vi "SubPanel_DataCollection_Rev11_v11.vi"(0 "DCPowerInformationClusterArray_Input":T7(array[cluster]), 1 "VISAPowerInfoInputArray":T6(array[cluster]), 2 "Run Data SubPanel Input":T5, 4 "Oscilloscope Info Array":T4(array[cluster]) {"vertical coupling" items=["AC", "DC", "Ground"]}, 6 "New Run?":bool, 7 "error in":errorcluster) -> (20 "DCPowerInformationClusterArray_Output":T7(array[cluster]), 21 "VISAPowerInfoInputOutput":T6(array[cluster]), 22 "Run Data SubPanel Output":T5, 23 "RF Block Parameters Output":T1, 24 "Oscilloscope Info Array Output":T4(array[cluster]) {"vertical coupling" items=["AC", "DC", "Ground"]}, 25 "Reinitialize?":bool, 26 "Data Was Collected?":bool, 27 "error out":errorcluster)   [LabVIEW 2019]
uses:
  Controls/DataBlockControl.ctl
  Controls/QueueDataControl_V3.ctl
  <vilib>/Utility/file.llb/Write Delimited Spreadsheet (string).vi
  Controls/RFBlockControl.ctl
  <instrlib>/niScope/Controls/niScope vertical coupling.ctl
panel:
  in  "RF Block Input Array":T1[](array[typedef])
  out "RFSourceInfoArray":string[][](array[string])
  out "OscilloscopeInfoArray":string[][](array[string])
  out "Voltage Waveform Array":waveform(dbl)[](array[waveform])
  out "Current Waveform Array":waveform(dbl)[](array[waveform])
  out "Current Measurements Live":T2(graph)
  out "Voltage Measurements Live":T2(graph)
  out "DCPowerInfoArray":string[][](array[string])
  out "Current Measurements Total":cluster{dbl[], dbl[]}[](graph)
  out "Voltage Measurements Total":cluster{dbl[], dbl[]}[](graph)
  out "Exiting":bool
  out "Full Run Information":string
  out "Ready For Next Run?":bool
  in  "Next Run":bool
  out "Recording Data":bool
  in  "Record Data Toggle":bool
  out "error of collection":errorcluster
  in  "force exit SubVI":bool
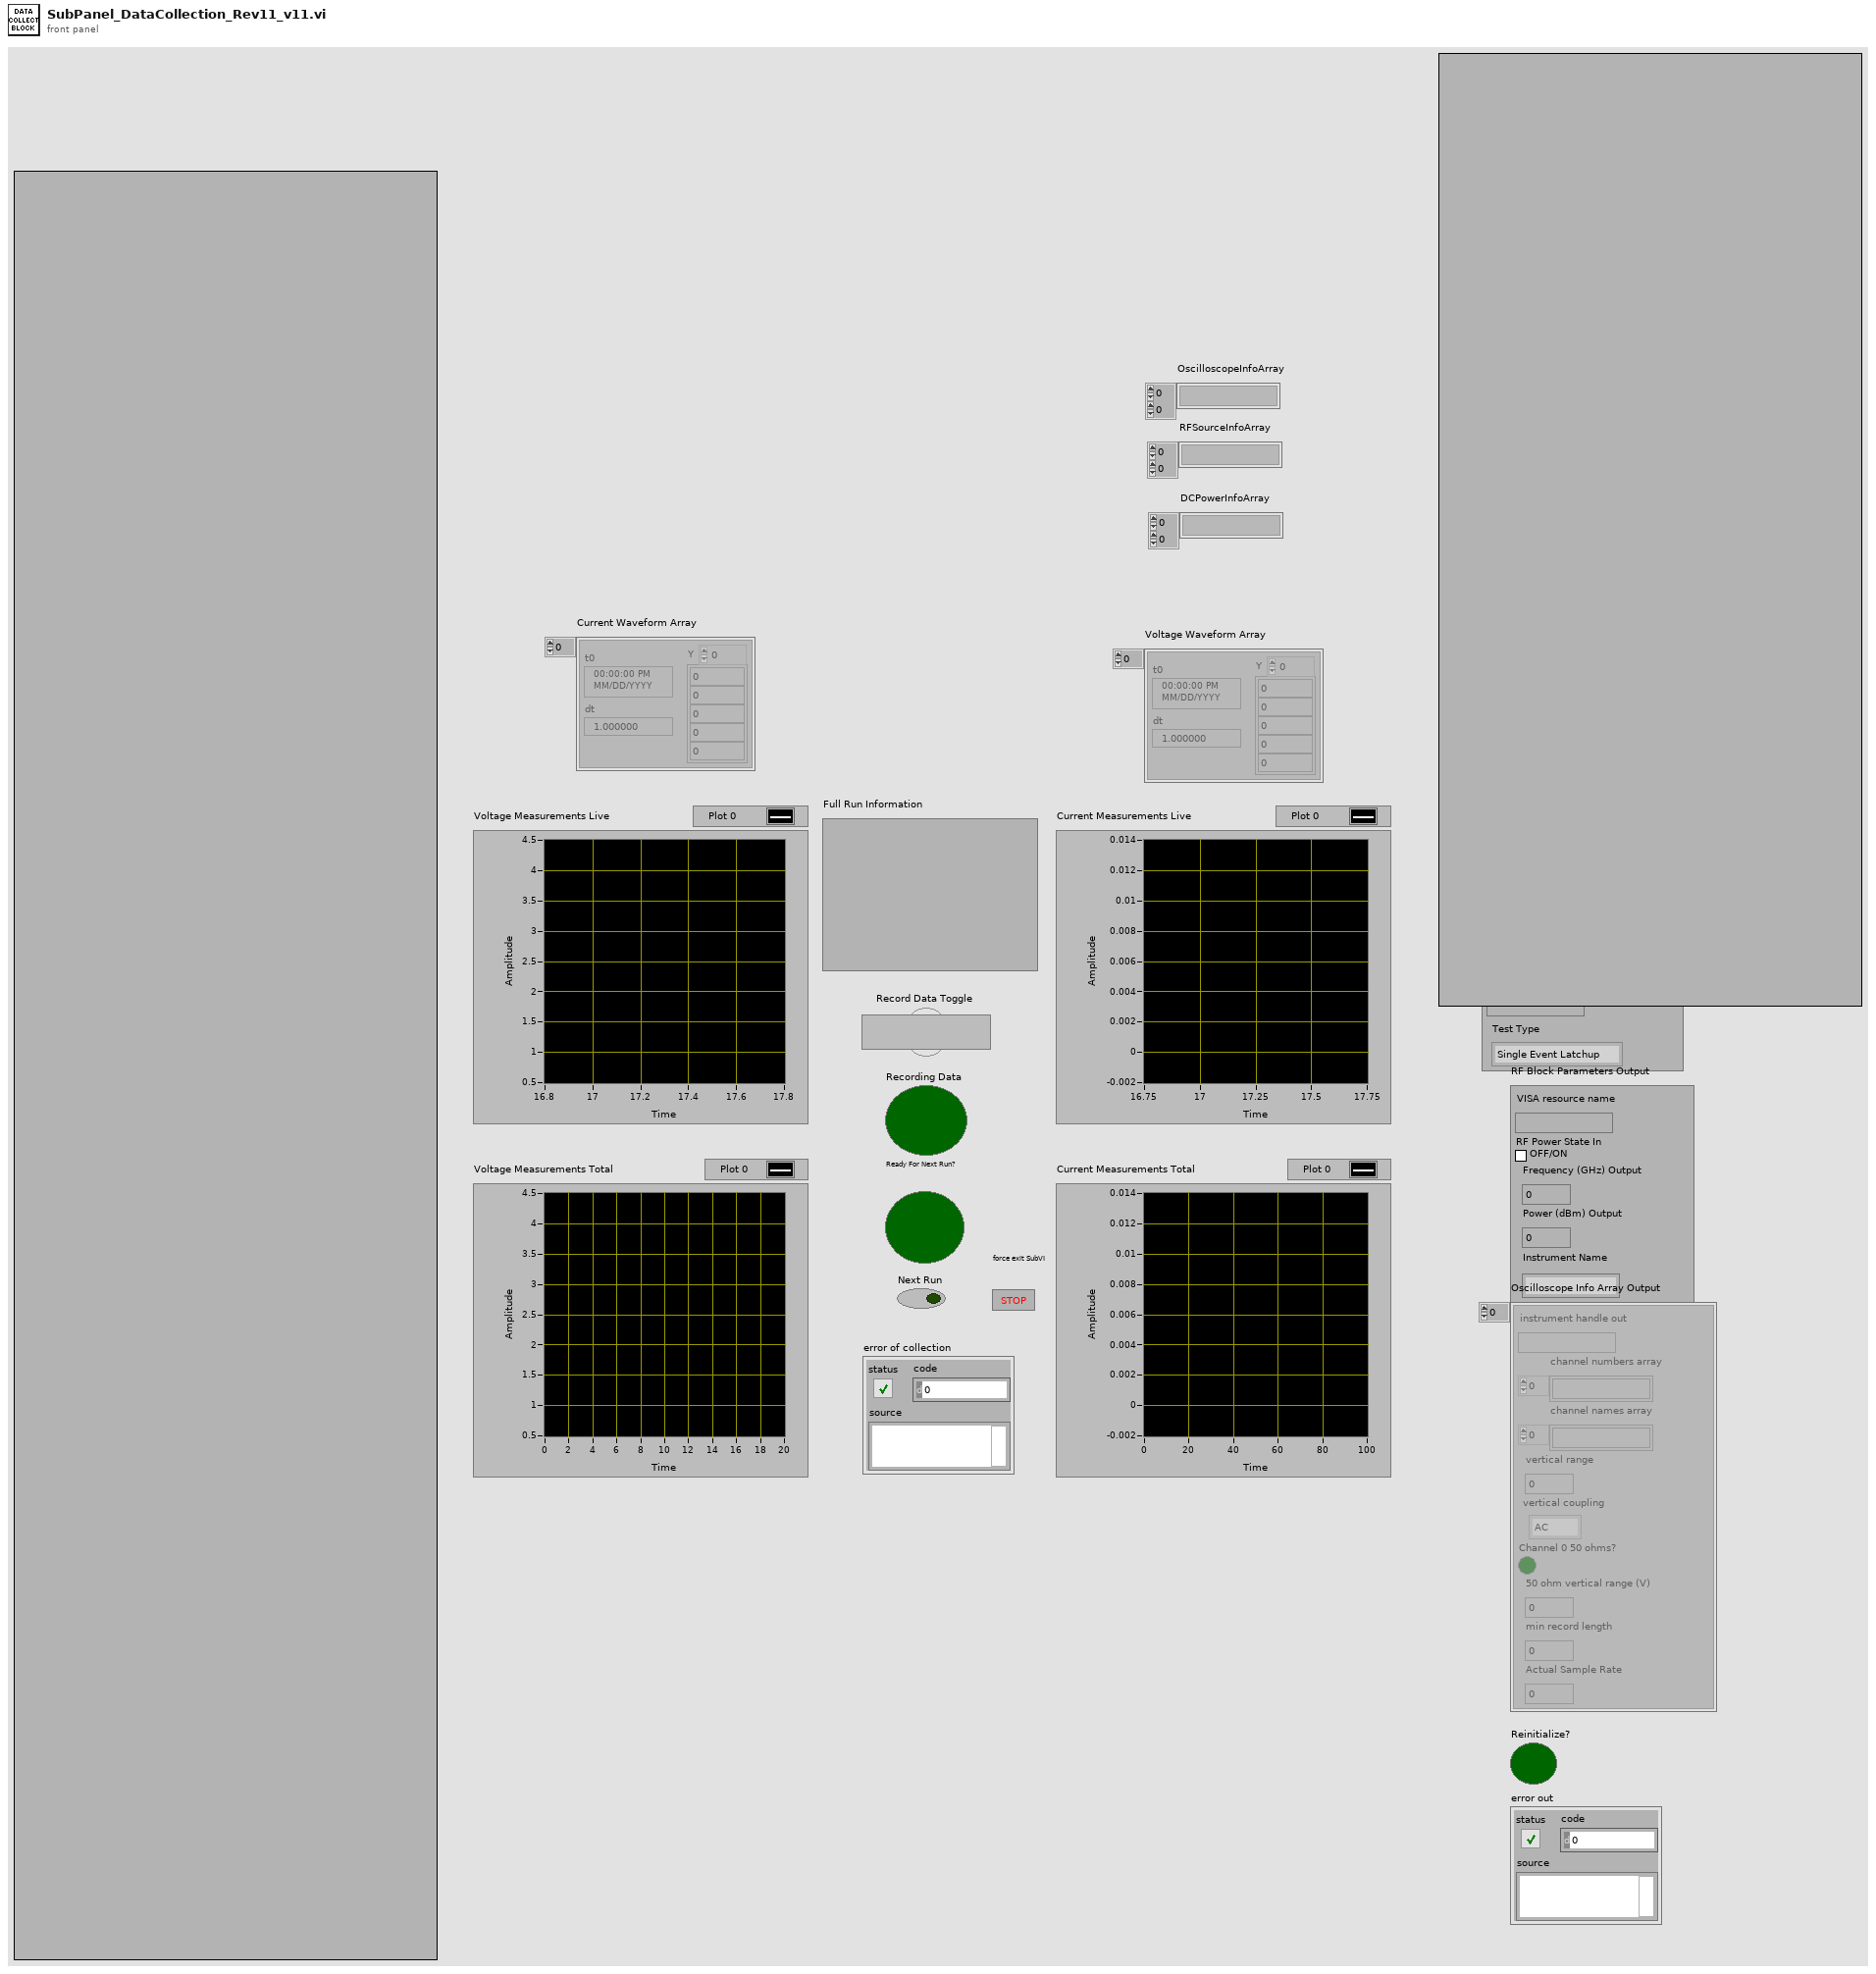
[diagram p1: front panel]
types:
  T1 = typedef "RFBlockControl.ctl" = cluster{"VISA resource name":refnum<visa-resource-name>, "RF Power State In":bool, "Frequency (GHz) Output":dbl, "Power (dBm) Output":dbl, "Instrument Name":string}
  T2 = cluster{"Array of fetched data":dbl[], "Array of fetched data":dbl[]}[]
  T3 = typedef "niScope vertical coupling.ctl" = i32
  T4 = cluster{"instrument handle out":refnum<k15>, "channel numbers array":string[], "channel names array":string[], "vertical range":dbl, "vertical coupling":T3, "Channel 0 50 ohms?":bool, "50 ohm vertical range (V)":dbl, "min record length":i32, "Actual Sample Rate":dbl}[]
  T5 = typedef "DataBlockControl.ctl" = cluster{"Run Folder Parent Directory":path, "DUT":string, "Ion (ex Kr)":string, "Board Number":string, "Effective LET":string, "Test Type":enum16{"Single Event Latchup", "Single Event Transient", "Single Event Upset"}}
  T6 = cluster{"VISA resource name":refnum<visa-resource-name>, "String List":string, string[], "Input Array (Voltage,Current_Limit)":dbl[], "Input Array (Voltage,Current_Limit)":dbl[], "Channel Names":string[], "read buffer":string}[]
  T7 = cluster{"instrument handle out":refnum<k15>, string, string[], dbl[], string[], "Current Limit Output Array":dbl[], dbl[]}[]
  T8 = enum16{"open", "replace", "create", "open or create", "replace or create", "replace or create with confirmation"}
  T9 = typedef "QueueDataControl_V3.ctl" = cluster{"Array of fetched data":dbl[][][], "Channel Names Array":string[], "Voltage Waveform Array":waveform(dbl)[], "Current Waveform Array":waveform(dbl)[], "Resetting Time":timestamp}
  T10 = cluster{"IVI Refnum out":refnum<k15>, string, "voltage level channel 23":dbl, "Channel Name 23":string, "Current Limit":dbl, "Measure Record dt":dbl, string}[]
  T11 = cluster{"created path":path, "DCPowerInformation_byChannel":cluster{"IVI Refnum out":refnum<k15>, string, "voltage level channel 23":dbl, "Channel Name 23":string, "Current Limit":dbl, "Measure Record dt":dbl, string}[], string[]}
  T12 = cluster{"Array of fetched data":dbl[][], string, i32[]}
  T13 = enum16{"Single Event Latchup", "Single Event Transient", "Single Event Upset"}
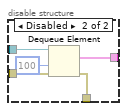
[diagram p2: hidden frame]
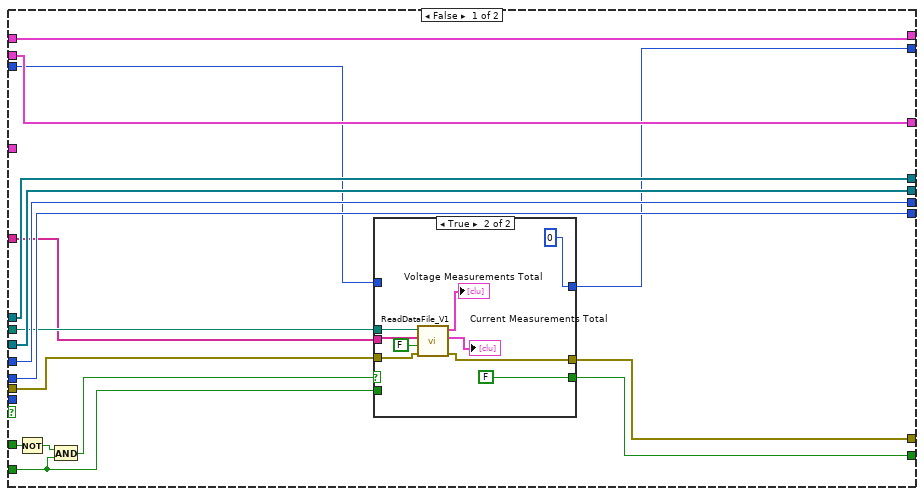
[diagram p3: hidden frame]
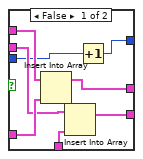
[diagram p5: hidden frame]
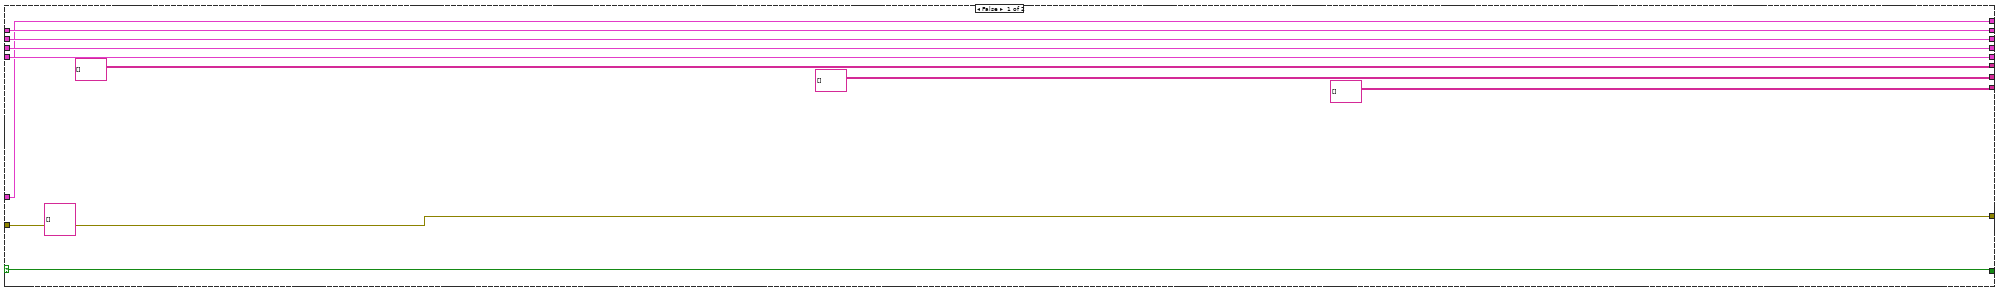
[diagram p6: hidden frame]
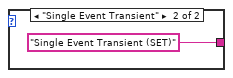
[diagram p7: hidden frame]
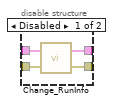
[diagram p11: hidden frame]
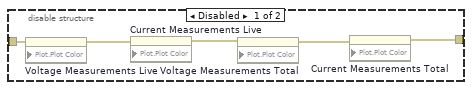
[diagram p12: hidden frame]
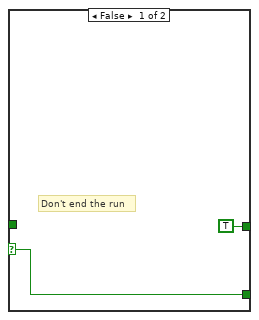
[diagram p14: hidden frame]
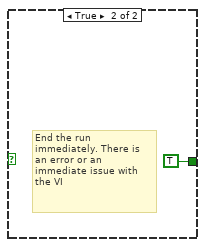
[diagram p15: hidden frame]
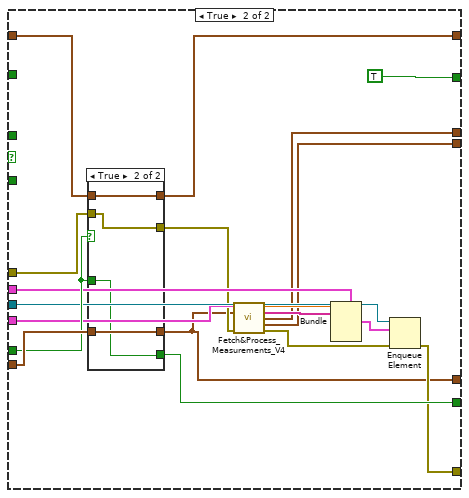
[diagram p18: hidden frame]
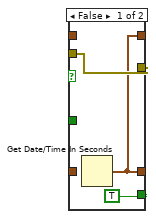
[diagram p19: hidden frame]
diagram:
  (unwired) string[] ["Instrument Name", "Channel Name", "Instrument Channel Number", "Voltage (V)", "Current Limit (A)", "Measure Record delta Time (s)"] ("new element/subarray")
  w76 = T9 {"Array of fetched data"=[], "Channel Names Array"=[], "Voltage Waveform Array"=[], "Current Waveform Array"=[], "Resetting Time"=timestamp(0 s since 1904-01-01)} ("DCPower Queue Data Double Array Format")
  (unwired) T9 {"Array of fetched data"=[], "Channel Names Array"=[], "Voltage Waveform Array"=[], "Current Waveform Array"=[], "Resetting Time"=timestamp(0 s since 1904-01-01)} ("DCPower Double Array Queue")
  (unwired) 10000 ("binary file indexor in")
  (unwired) T5 {"Run Folder Parent Directory"=path "", "DUT"="", "Ion (ex Kr)"="", "Board Number"="", "Effective LET"="", "Test Type"=enum."Single Event Latchup"} ("Run Data Configuration")
  # "Initiating the queue"
  # "echoing run information"
  # "Checking if this is a new run. If it is, a new folder is created along with references to a datafile node. If it is not new (i.e. you didn't start recording data because you needed to make a last minute change and pressed forced exit subvi), the previous folder that is theoretically empty (or just has the .txt files is used"
  # "If yes, you go into this subVI"
  # "This is the message at the beginning confirming if you want to make small changes to the program (i.e. LET)"
  # "Parameters from the configuration stage of this program"
  # "Reset the graph that is saving every 10 seconds of data. Every reset the low bound of the ten seconds is"
  # "Need to change to reflect number of channels that are being recorded. Collect this from a parameters file eventually that will be created"
  # "Indicator if the system is ready for another run. Also indicates if data was actually collected"
  # "Resets the system to start recording"
  # "A flag to ensure the warning message shows only once and doesn't lock the system"
  # "Initiating all of the DC Power instruments (doing this here so because we force abort channels in the DCPower setup because buffer overflow issues. Iterating over the instrument array and the active channel list"
  n1 = flat-sequence {
    tunnel: [w117] -> w92
    tunnel: "error in" -> [w107]
    tunnel: [w121] -> w97
    tunnel: "Run Data SubPanel Input" -> [w109]
    frame #0 {
      n2 = disable-structure shown="Enabled" {
        disable-tunnel: w107 -> [w126 w127]
        disable-tunnel: [w122 w127] -> w106
        frame Disabled {
          n3 = property on="Voltage Measurements Live" class="XYGraph (strict)" props=["Plot", "Plot Color"](error in=w126) -> (error out=w125:errorcluster)  [unwired: 2 in, 1 out]
          n4 = property on="Current Measurements Live" class="XYGraph (strict)" props=["Plot", "Plot Color"](error in=w125) -> (error out=w124:errorcluster)  [unwired: 2 in, 1 out]
          n5 = property on="Voltage Measurements Total" class="XYGraph (strict)" props=["Plot", "Plot Color"](error in=w124) -> (error out=w123:errorcluster)  [unwired: 2 in, 1 out]
          n6 = property on="Current Measurements Total" class="XYGraph (strict)" props=["Plot", "Plot Color"](error in=w123) -> (error out=w122:errorcluster)  [unwired: 2 in, 1 out]
        }
        frame Enabled {
        }
      }
      n7 = local write "Voltage Measurements Total"(cluster{dbl[], dbl[]}[] [] ("Voltage Measurements")) -> ()
      n8 = local write "Current Measurements Total"(cluster{dbl[], dbl[]}[] [] ("Current Measurements")) -> ()
      n9 = local write "Recording Data"(FALSE ("Recording Data")) -> ()
      n10 = local write "Exiting"(FALSE ("Forced Exit")) -> ()
      n11 = call "Convert_RunInfoCluster_2_RunInfoStringList.vi"("error in"=w106, "Run Number"="", "Run Data SubPanel Input"=w109) -> ("error output"=w110:errorcluster, "Run Data Output"=w111:string)
      n12 = call "Display Message to User"("error in (no error)"=w110, "Enable"=TRUE, "Message"=w111) -> ("error out"=w117:errorcluster)  [unwired: 7 in, 1 out]
      n13 = Two Button Dialog(message="Changing the LET?", 1:"No" ("F button name (\"Cancel\")"), 2:"Yes" ("T button name (\"OK\")")) -> (T button?=w121:bool)
    }
  }
  n14 = call "Convert_InstrumentReferenceArray_2_ChannelReferenceArray.vi"("error in (no error)"=w92, "DCPowerInformationClusterArray_Input"="DCPowerInformationClusterArray_Input") -> ("error out"=w91:errorcluster, "DCPowerInformation_byChannel"=w51:T10)
  n15 = case shown="True" w97 {
    tunnel: "Run Data SubPanel Input" -> [w129 w133]
    tunnel: [w129 w132] -> w29
    tunnel: [w128 w131] -> w93
    tunnel: w91 -> [w128 w130]
    frame False {
    }
    frame True {
      n16 = disable-structure shown="Enabled" {
        disable-tunnel: w133 -> [w137 w139]
        disable-tunnel: [w136 w138] -> w132
        disable-tunnel: [w135 w141] -> w131
        disable-tunnel: w130 -> [w134 w140]
        frame Disabled {
          n17 = call "Change_RunInfo.vi"("error in (no error)"=w134, "Run Data SubPanel in"=w137) -> ("error out"=w135:errorcluster, "Run Data SubPanel out"=w136:T5)
        }
        frame Enabled {
          n18 = call "Change_RunInfo_V2.vi"("error in (no error)"=w140, "Run Data SubPanel in"=w139) -> ("error out"=w141:errorcluster, "Run Data SubPanel out"=w138:T5)
        }
      }
    }
  }
  n19 = Unbundle(w29) -> ("Run Folder Parent Directory"=w94:path)  [unwired: 5 out]
  n20 = List Folder(path=w94, error in=w93) -> (folder names=w95:string[], error out=w79:errorcluster)  [unwired: 2 in, 2 out]
  n21 = Array Size(array=w95) -> (size(s)=w82:i32)
  n22 = case shown="True" "New Run?" {
    selector: "New Run?" -> [w143 w146]
    tunnel: [w144 w148] -> w83
    tunnel: w82 -> [w144 w147]
    tunnel: [w143 w146] -> w81
    tunnel: [w142 w145] -> w80
    tunnel: w79 -> [w142 w145]
    frame False {
    }
    frame True {
      n23 = Increment(x=w147) -> (x+1=w148:i32)
    }
  }
  n24 = Number To Decimal String(number=w83) -> (decimal integer string=w86:string)  [unwired: 1 in]
  n25 = Concatenate Strings("Run_", w86) -> (w28:string)
  n26 = Array Size(array=w51) -> (size(s)=w78:i32)
  n27 = call "InitialFileFolderCreation_V2.vi"("New Run?"=w81, "error in (no error)"=w80, "Run Number"=w28, "DCPowerArrayClusterSize"=w78, "base path"=w94) -> ("error out"=w27:errorcluster, "SupplementalDataFileReferenceObjectArray"=w89:refnum<file>[], "DataFileReferenceObjectArray"=w90:refnum<file>[], "created path"=w36:path)  [unwired: 3 in]
  n28 = call "Convert_RunInfoCluster_2_RunInfoStringList.vi"("error in"=w27, "Run Number"=w28, "Run Data SubPanel Input"=w29) -> ("error output"=w26:errorcluster, "Run Data Output"=→"Full Run Information":string)
  n29 = for {
    shift-right: [w149] -> w34
    shift-left: w26 -> [w151]
    tunnel: "DCPowerInformationClusterArray_Input" -> [w153] mode=indexing
    n30 = Unbundle(w153) -> ("instrument handle out"=w150:refnum<k15>, w152:string)  [unwired: 5 out]
    n31 = call <instrlib>:"niDCPower Initiate With Channels.vi"("error in (no error)"=w151, "channel name"=w152, "instrument handle"=w150) -> ("error out"=w149:errorcluster)  [unwired: 7 in, 1 out]
  }
  n32 = disable-structure shown="Enabled" {
    disable-tunnel: w34 -> [w157 w159]
    disable-tunnel: [w156 w159] -> w31
    disable-tunnel: [w155 _] -> w102
    disable-tunnel: w76 -> [w154 _]
    frame Enabled {
      n33 = Obtain Queue(name (unnamed)="DCPowerQueue", element data type=w154, error in (no error)=w157) -> (queue out=w155:refnum<queue>, error out=w156:errorcluster)  [unwired: 2 in, 1 out]
    }
    frame Disabled {
    }
  }
  n34 = for {
    tunnel: w51 -> [w161] mode=indexing
    tunnel: [w160] -> w52 mode=indexing
    # "Creating Array of Channel Names"
    n35 = Unbundle(w161) -> ("Channel Name 23"=w160:string)  [unwired: 6 out]
  }
  n36 = Bundle("created path"=w36, "DCPowerInformation_byChannel"=w51, w52) -> (w50:T11)  [unwired: 1 in]
  n37 = Array Size(array=w52) -> (size(s)=w71:i32)
  n38 = Get Date/Time In Seconds() -> (seconds since 1Jan1904=w32:timestamp)
  n39 = while {
    shift-right: [w192] -> w40
    shift-left: "DCPowerInformationClusterArray_Input" -> [w192]
    shift-right: [w196] -> w42
    shift-left: "VISAPowerInfoInputArray" -> [w196]
    shift-right: [w195] -> w44
    shift-left: w29 -> [w195]
    shift-right: [w194] -> w46
    shift-left: "RF Block Input Array" -> [w194]
    shift-right: [w193] -> w48
    shift-left: "Oscilloscope Info Array" -> [w193]
    shift-right: [w179] -> w77
    shift-left: w31 -> [w190]
    tunnel: w51 -> [w191]
    shift-right: [w189] -> _
    shift-left: FALSE -> [w186]
    tunnel: w102 -> [w188]
    shift-right: [w168] -> _
    shift-left: FALSE -> [w173]
    tunnel: [w177] -> w101
    shift-right: [w171] -> _
    shift-left: TRUE ("x .and. y?") -> [w172]
    shift-right: [w169] -> _
    shift-left: w32 -> [w170]
    tunnel: [w168] -> w39
    tunnel: w76 -> [w166]
    shift-right: [w163] -> w19
    shift-left: timestamp(0 s since 1904-01-01) ("seconds since 1Jan1904") -> [w162]
    stop <- w167 stop-if-true
    # "If I am going to reset the entire configuration or if we are going up in LET only. True, reset the system. False, don't reset the system"
    n40 = Not(x=w173) -> (.not. x?=w175:bool)
    n41 = And(x="Record Data Toggle", y=w175) -> (x .and. y?=w176:bool)
    "Recording Data" <- w176
    n42 = case shown="False" w176 {
      tunnel: w191 -> [w225 w240]
      tunnel: w190 -> [w223 w247]
      tunnel: [w213 w235] -> w165
      tunnel: [w214 w234] -> w164
      tunnel: w186 -> [_ w245]
      tunnel: [FALSE w246] -> w189
      tunnel: w188 -> [_ w244]
      tunnel: [w212 w243] -> w184
      tunnel: "Record Data Toggle" -> [w220 _]
      tunnel: w173 -> [w221 _]
      tunnel: w172 -> [w216 _]
      tunnel: [w217 TRUE] -> w171
      tunnel: w170 -> [w215 w248]
      tunnel: [w215 w238] -> w169
      tunnel: w166 -> [_ w242]
      tunnel: [w211 w232] -> w163
      tunnel: w162 -> [w211 w231]
      frame False {
        n43 = And(x=w220, y=w221) -> (x .and. y?=w219:bool)
        n44 = And(x=w216, y=w219) -> (x .and. y?=w218:bool)
        n45 = case shown="True" w218 {
          tunnel: [w227 w229] -> w222
          tunnel: w223 -> [w227 w230]
          tunnel: [w226 FALSE] -> w217
          tunnel: w216 -> [w226 _]
          frame False {
          }
          frame True {
            n46 = call "Display Message to User2"("error in (no error)"=w230) -> ("error out"=w229:errorcluster)  [unwired: 9 in, 1 out]
          }
        }
        n47 = call "Fetch&Process_Measurements_V4.vi"("DCPowerInformation_byChannel"=w225, "Initial Time"=w215, "error in (no error)"=w222) -> ("Current Waveform Array"=w213:waveform(dbl)[], "Voltage Waveform Array"=w214:waveform(dbl)[], "error out"=w212:errorcluster)  [unwired: 6 in, 4 out]
      }
      frame True {
        n48 = case shown="True" w245 {
          tunnel: [w250 w256] -> w238
          tunnel: w248 -> [_ w256]
          tunnel: w247 -> [w251 w255]
          tunnel: [w251 w255] -> w239
          tunnel: [TRUE w254] -> w246
          tunnel: w245 -> [_ w254]
          tunnel: [w250 w253] -> w232
          tunnel: w231 -> [_ w253]
          frame False {
            n49 = Get Date/Time In Seconds() -> (seconds since 1Jan1904=w250:timestamp)
          }
          frame True {
          }
        }
        n50 = call "Fetch&Process_Measurements_V4.vi"("DCPowerInformation_byChannel"=w240, "Initial Time"=w238, "error in (no error)"=w239) -> ("Data As dbl Array"=w237:dbl[][][], "Channel Number Array"=w236:string[], "Current Waveform Array"=w235:waveform(dbl)[], "Voltage Waveform Array"=w234:waveform(dbl)[], "error out"=w233:errorcluster)  [unwired: 6 in, 2 out]
        n51 = Bundle(cluster=w242, "Array of fetched data"=w237, "Channel Names Array"=w236) -> (w241:T9)  [unwired: 3 in]
        n52 = Enqueue Element(queue=w244, element=w241, error in (no error)=w233) -> (error out=w243:errorcluster)  [unwired: 1 in, 2 out]
      }
    }
    "Current Waveform Array" <- w165
    "Voltage Waveform Array" <- w164
    n53 = Not(x=w176) -> (.not. x?=w187:bool)
    n54 = And(x=w187, y=w186) -> (x .and. y?=w185:bool)
    n55 = case shown="True" w185 {
      tunnel: w184 -> [w207 w209]
      tunnel: [w208 TRUE] -> w168
      tunnel: w173 -> [w208 _]
      tunnel: [w207 w209] -> w179
      frame False {
      }
      frame True {
      }
    }
    "error of collection" <- w179
    "Ready For Next Run?" <- w168
    n56 = Or(x=w179, y="force exit SubVI") -> (x .or. y?=w181:bool)
    n57 = And(x="Next Run", y=w168) -> (x .and. y?=w183:bool)
    n58 = Or(x=w181, y=w183) -> (x .or. y?=w182:bool)
    n59 = case shown="True" w182 {
      selector: w182 -> [w198 _]
      tunnel: w181 -> [_ w201]
      tunnel: [w198 TRUE] -> w167
      tunnel: [TRUE ("T button?") w199] -> w177
      frame False {
        # "Don't end the run"
      }
      frame True {
        n60 = case shown="False" w201 {
          tunnel: [w202 TRUE] -> w199
          frame False {
            # "Option to continue the run as is or reset for a new configuration"
            n61 = Two Button Dialog(message="Would you like to change parameters before the next run? ( you will have an option to change LET and board number regardless) ", 1:"No, I may only want to change LET or board number" ("F button name (\"Cancel\")"), 2:"Yes, I want to make changes " ("T button name (\"OK\")")) -> (T button?=w202:bool)
          }
          frame True {
            # "End the run immediately. There is an error or an immediate issue with the VI"
          }
        }
      }
    }
    "Exiting" <- w167
  }
  "Reinitialize?" <- w101
  n62 = while {
    tunnel: w102 -> [w289]
    shift-right: [w276] -> w73
    shift-left: w31 -> [w288]
    tunnel: w36 -> [w285]
    shift-right: [w278] -> w75
    shift-left: w90 -> [w286]
    shift-right: [w277] -> w74
    shift-left: w89 -> [w284]
    shift-right: [w280] -> _
    shift-left: 0 ("binary file indexor in") -> [w283]
    shift-right: [w279] -> _
    shift-left: 0 ("binary file indexor in") -> [w282]
    tunnel: 1000 ("binary file indexor in") -> [w281]
    tunnel: w52 -> [w287]
    tunnel: w71 -> [_]
    shift-right: [w265] -> _
    shift-left: FALSE -> [w264]
    shift-right: [w261] -> _
    shift-left: T2 [] ("array") -> [w262]
    shift-right: [w259] -> _
    shift-left: T2 [] ("array") -> [w260]
    shift-right: [w257] -> _
    shift-left: 0 -> [w258]
    stop <- w273 stop-if-true
    # "If recording data is on, there should always be elements in the queue, so I shouldn't have to worry about a state where the \"recording data\" is active but there is no data in the queue, if so, then I'll just have to find an alternative to the OR statement"
    n63 = Get Queue Status(queue=w289, error in (no error)=w288) -> (queue out=w270:refnum<queue>, error out=w271:errorcluster, # elements in queue=w266:i32)  [unwired: 1 in, 5 out]
    n64 = local read "Recording Data"() -> (w263:bool)
    n65 = disable-structure shown="Enabled" {
      disable-tunnel: [w293 w295] -> w272
      disable-tunnel: w271 -> [w292 w297]
      disable-tunnel: w270 -> [w291 w298]
      disable-tunnel: [w290 w294] -> w269
      frame Enabled {
        n66 = Flush Queue(queue=w291, error in (no error)=w292) -> (remaining elements=w290:T9[], error out=w293:errorcluster)  [unwired: 1 out]
      }
      frame Disabled {
        n67 = Dequeue Element(queue=w298, timeout in ms (-1)=100, error in (no error)=w297) -> (element=w294:T9, error out=w295:errorcluster)  [unwired: 2 out]
      }
    }
    n68 = Not Equal To 0?(x=w266) -> (x != 0?=w268:bool)
    n69 = And(x=w268, y=w263) -> (x .and. y?=w267:bool)
    n70 = case shown="True" w267 {
      tunnel: w269 -> [_ w355]
      tunnel: w272 -> [w306 w349]
      tunnel: w287 -> [w307 w341]
      tunnel: w286 -> [w314 w354]
      tunnel: w285 -> [w308 w353]
      tunnel: w284 -> [w315 w352]
      tunnel: w283 -> [w313 w351]
      tunnel: w282 -> [w312 w340]
      tunnel: w281 -> [_ w339]
      tunnel: [w313 w348] -> w280
      tunnel: [w312 w347] -> w279
      tunnel: [w314 w344] -> w278
      tunnel: [w315 w343] -> w277
      tunnel: [w305 w342] -> w276
      tunnel: [w304 TRUE] -> w265
      tunnel: w264 -> [w303 _]
      tunnel: w263 -> [w311 _]
      tunnel: w262 -> [w302 w335]
      tunnel: [w302 w334] -> w261
      tunnel: w260 -> [w301 w333]
      tunnel: [w301 w332] -> w259
      tunnel: w258 -> [w300 w329]
      tunnel: [w299 w328] -> w257
      frame False {
        n71 = Not(x=w311) -> (.not. x?=w310:bool)
        n72 = And(x=w310, y=w303) -> (x .and. y?=w309:bool)
        n73 = case shown="True" w309 {
          tunnel: w308 -> [_ w327]
          tunnel: w307 -> [_ w326]
          tunnel: w306 -> [w318 w324]
          tunnel: [w318 w323] -> w305
          tunnel: [w317 FALSE] -> w304
          tunnel: w303 -> [w317 _]
          tunnel: w300 -> [w316 _]
          tunnel: [w316 0] -> w299
          frame False {
          }
          frame True {
            n74 = call "ReadDataFile_V1.vi"("error in (no error)"=w324, "Create CSV files?"=FALSE, "Channel Names Array"=w326, "DataFolder Path"=w327) -> ("error out"=w323:errorcluster, "Current Measurements"=→"Current Measurements Total":cluster{dbl[], dbl[]}[], "Voltage Measurements"=→"Voltage Measurements Total":cluster{dbl[], dbl[]}[])  [unwired: 5 in]
          }
        }
      }
      frame True {
        # "structure where each channel has its own data and supplemental file. Intent for faster data reading speeds in post processing. Probably not since would be i^3, but if we used multiple cores, maybe it would be advantageous"
        n75 = call "FilePathCreation_DCPower_V2.vi"("binary file input reference array 1"=w354, "Channel Name Input array"=w341, "data output directory folder"=w353, "binary file indexor in"=w351, "Reset counter in"=w340, "error in (no error)"=w349, "binary file input reference array 2"=w352, "reset threshold"=w339) -> ("binary file output reference array"=w346:refnum<file>[], "binary file output reference array 2"=w345:refnum<file>[], "binary file indexor out"=w348:i32, "reset counter out"=w347:i32, "error out"=w350:errorcluster)  [unwired: 3 in]
        n76 = for {
          shift-right: [w380] -> w342
          shift-left: w350 -> [w381]
          tunnel: w355 -> [w390]
          tunnel: w345 -> [w387] mode=indexing
          tunnel: w346 -> [w386] mode=indexing
          tunnel: [w385] -> w343 mode=indexing
          tunnel: [w379] -> w344 mode=indexing
          tunnel: [w374] -> w337 mode=indexing
          tunnel: [w373] -> w336 mode=indexing
          i -> [w384]
          n77 = for {
            tunnel: w390 -> [w403] mode=indexing
            tunnel: w384 -> [w400]
            tunnel: [w395] -> w375 mode=concatenating
            tunnel: [w399] -> w389
            tunnel: w387 -> [w398]
            tunnel: w386 -> [w396]
            tunnel: [w396] -> w382
            tunnel: [w398] -> w385
            tunnel: [w397] -> w388 mode=concatenating
            n78 = Unbundle(w403) -> ("Array of fetched data"=w402:dbl[][][], "Channel Names Array"=w401:string[])  [unwired: 3 out]
            n79 = Index Array(array=w401, index=w400) -> (element=w399:string)
            n80 = Index Array(array=w402, index (dim 0)=w400) -> (element=w395:dbl[][])  [unwired: 2 in]
            n81 = Array Size(array=w395) -> (size(s)=w397:i32[])
          }
          n82 = Bundle("Array of fetched data"=w375, w389, w388) -> (w383:T12)  [unwired: 1 in]
          n83 = Index Array(array=w375, index (row)=2) -> (element=w368:dbl[])  [unwired: 1 in]
          n84 = Index Array(array=w375, index (row)=1) -> (element=w370:dbl[])  [unwired: 1 in]
          n85 = Index Array(array=w375, index (row)=0) -> (element=w372:dbl[])  [unwired: 1 in]
          n86 = call "DataFileNode_Entry_V4.vi"("error in (no error)"=w381, "Queued Elements"=w383, "Byte Stream File in"=w382) -> ("error out"=w380:errorcluster, "Byte Stream File out"=w379:refnum<file>)  [unwired: 7 in]
          n87 = for {
            tunnel: [w392] -> w367 mode=indexing if=w391
            tunnel: w372 -> [w392] mode=indexing
            tunnel: [w394] -> w371 mode=indexing if=w391
            tunnel: w370 -> [w394] mode=indexing
            tunnel: [w393] -> w369 mode=indexing if=w391
            tunnel: w368 -> [w393] mode=indexing
            n88 = Not Equal To 0?(x=w392) -> (x != 0?=w391:bool)
          }
          n89 = Bundle(w367, w371) -> (w374:cluster{dbl[], dbl[]})  [unwired: 1 in]
          n90 = Bundle(w367, w369) -> (w373:cluster{dbl[], dbl[]})  [unwired: 1 in]
        }
        n91 = Greater?(x=w329, y=99) -> (0:w331:bool)
        n92 = case shown="True" w331 {
          tunnel: w337 -> [w363 _]
          tunnel: w336 -> [w362 _]
          tunnel: w335 -> [w361 _]
          tunnel: [w360 T2 [] ("array")] -> w334
          tunnel: w333 -> [w359 _]
          tunnel: [w358 T2 [] ("array")] -> w332
          tunnel: w329 -> [w357 _]
          tunnel: [w356 0] -> w328
          frame False {
            n93 = Insert Into Array(array=w361, new element=w363) -> (w360:T2)  [unwired: 1 in]
            n94 = Insert Into Array(array=w359, new element=w362) -> (w358:T2)  [unwired: 1 in]
            n95 = Increment(x=w357) -> (x+1=w356:i32)
          }
          frame True {
          }
        }
        "Voltage Measurements Live" <- w334
        "Current Measurements Live" <- w332
      }
    }
    n96 = local read "Exiting"() -> (w275:bool)
    n97 = Equal To 0?(x=w266) -> (x = 0?=w274:bool)
    n98 = And(x=w274, y=w275) -> (x .and. y?=w273:bool)
  }
  n99 = for {
    tunnel: w75 -> [w408] mode=indexing
    tunnel: w74 -> [w406] mode=indexing
    shift-right: [w404] -> w72
    shift-left: w73 -> [w407]
    n100 = Close File(refnum=w408, error in=w407) -> (error out=w405:errorcluster)  [unwired: 1 out]
    n101 = Close File(refnum=w406, error in=w405) -> (error out=w404:errorcluster)  [unwired: 1 out]
  }
  n102 = Merge Errors(w77, w72) -> (w54:errorcluster)
  n103 = Unbundle(w50) -> ("created path"=w35:path)  [unwired: 2 out]
  n104 = case shown="True" w39 {
    selector: w39 -> [w413 w518]
    tunnel: w54 -> [w412 w524]
    tunnel: [w412 w423] -> w53
    tunnel: [w418 w455] -> w49
    tunnel: w48 -> [w418 w523]
    tunnel: [w417 w457] -> w47
    tunnel: w46 -> [w417 w522]
    tunnel: [w416 w443] -> w45
    tunnel: w44 -> [w416 w521]
    tunnel: [w415 w460] -> w43
    tunnel: w42 -> [w415 w520]
    tunnel: [w414 w462] -> w41
    tunnel: w40 -> [w414 w519]
    tunnel: [w413 w518] -> w38
    tunnel: [string[][] [] ("DCPowerInfoArray") w453] -> w37
    tunnel: w35 -> [_ w421]
    tunnel: [string[][] [] ("DCPowerInfoArray") w451] -> w3
    tunnel: [string[][] [] ("DCPowerInfoArray") w445] -> w2
    frame False {
      (unwired) string[][][] []
    }
    frame True {
      # "This will be indexed eventually"
      n105 = for {
        shift-right: [w604] -> w514
        shift-left: w524 -> [w616]
        tunnel: w519 -> [w607] mode=indexing
        shift-right: [w615] -> w493
        shift-left: w523 -> [w615]
        shift-right: [w614] -> w492
        shift-left: w522 -> [w614]
        shift-right: [w613] -> w491
        shift-left: w521 -> [w613]
        shift-right: [w612] -> w490
        shift-left: w520 -> [w612]
        shift-right: [w611] -> w489
        shift-left: w519 -> [w611]
        shift-right: [w609] -> w494
        shift-left: string[][] [] ("DCPowerInfoArray") -> [w610]
        # "This puts all the instruments together in one output"
        n106 = Unbundle(w607) -> ("instrument handle out"=w618:refnum<k15>, w617:string)  [unwired: 5 out]
        n107 = call <instrlib>:"niDCPower Abort With Channels.vi"("error in (no error)"=w616, "channel name"=w617, "instrument handle"=w618) -> ("error out"=w605:errorcluster)  [unwired: 7 in, 1 out]
        n108 = call "DCPower_ParameterCreation.vi"("error in"=w605, "Precision"="8", "DCPowerInformationByInstrument"=w607) -> ("error out"=w604:errorcluster, "DCPowerInfoArray"=w603:string[][])
        n109 = Insert Into Array(array=w610, index (col)=0 ("disabled index (col)"), new element=w603) -> (w609:string[][])  [unwired: 1 in]
      }
      n110 = Concatenate Strings("Channel Name " ("string")) -> (w506:string)
      n111 = Concatenate Strings("Voltage (V) " ("string")) -> (w508:string)
      n112 = Concatenate Strings("Measure Record delta Time (s) " ("string")) -> (w510:string)
      n113 = Concatenate Strings("Instrument Name " ("string")) -> (w505:string)
      n114 = Concatenate Strings("Instrument Channel Number " ("string")) -> (w507:string)
      n115 = Concatenate Strings("Current Limit (A) " ("string")) -> (w509:string)
      n116 = Build Array(w505, w506, w507, w508, w509, w510) -> (w498:string[])
      n117 = Build Path(base path=w421, name or relative path="DCPOW_Params.csv") -> (appended path=w513:path)
      n118 = Insert Into Array(array=w494, index (col)=0 ("disabled index (col)"), new element=w498) -> (w497:string[][])  [unwired: 1 in]
      n119 = call-poly <vilib>:"Write Delimited Spreadsheet.vi"("file path (dialog if empty)"=w513, "format (%s)"="%s" ("format (%.3f)"), "2D data"=w497, "error in (no error)"=w514, "transpose? (no:F)"=TRUE, "delimiter (\\t)"="," ("delimiter (\\t)")) -> ("error out"=w495:errorcluster)  [unwired: 8 in, 1 out]
      n120 = for {
        shift-right: [w597] -> w475
        shift-left: w495 -> [w597]
        shift-right: [w592] -> w463
        shift-left: w489 -> [w592]
        shift-right: [w593] -> w461
        shift-left: w490 -> [w593]
        shift-right: [w594] -> w459
        shift-left: w491 -> [w594]
        shift-right: [w595] -> w458
        shift-left: w492 -> [w595]
        shift-right: [w596] -> w454
        shift-left: w494 -> [w596]
        tunnel: w493 -> [w591] mode=indexing
        tunnel: [w591] -> w456 mode=indexing
        shift-right: [w560] -> w452
        shift-left: string[][] [] ("DCPowerInfoArray") -> [w566]
        n121 = Unbundle(w591) -> ("instrument handle out"=w590:refnum<k15>, "channel numbers array"=w563:string[], "channel names array"=w564:string[], "vertical range"=w585:dbl, "vertical coupling"=w579:T3, "Channel 0 50 ohms?"=w584:bool, "50 ohm vertical range (V)"=w583:dbl, "min record length"=w578:i32, "Actual Sample Rate"=w577:dbl)
        n122 = Array Size(array=w563) -> (size(s)=w586:i32)
        n123 = Initialize Array(w585, w586) -> (w582:dbl[])
        n124 = Decimal String To Number(string="8") -> (number=w561:i32)  [unwired: 2 in, 1 out]
        n125 = case shown="True" w584 {
          tunnel: w583 -> [_ w600]
          tunnel: w582 -> [w598 w602]
          tunnel: [w598 w599] -> w581
          frame False {
          }
          frame True {
            n126 = Replace Array Subset(array=w602, new element=w600, index=0) -> (w599:dbl[])
          }
        }
        n127 = Number To Fractional String(number=w577, precision (6)=w561) -> (F-format string=w571:string)  [unwired: 2 in]
        n128 = Number To Decimal String(number=w578) -> (decimal integer string=w572:string)  [unwired: 1 in]
        n129 = Concatenate Strings(w590) -> (w588:string)
        n130 = Number To Fractional String(number=w581, precision (6)=w561) -> (F-format string=w580:string[])  [unwired: 2 in]
        n131 = Number To Decimal String(number=w579) -> (decimal integer string=w573:string)  [unwired: 1 in]
        n132 = Array Size(array=w563) -> (size(s)=w589:i32)
        n133 = Initialize Array(w588, w589) -> (w587:string[])
        n134 = Array Size(array=w563) -> (size(s)=w576:i32)
        n135 = Array Size(array=w563) -> (size(s)=w574:i32)
        n136 = Array Size(array=w563) -> (size(s)=w575:i32)
        n137 = Initialize Array(w573, w576) -> (w570:string[])
        n138 = Initialize Array(w571, w574) -> (w568:string[])
        n139 = Initialize Array(w572, w575) -> (w569:string[])
        n140 = Build Array(w587, w564, w563, w580, w570, w569, w568) -> (w565:string[][])
        n141 = Insert Into Array(array=w566, index (col)=0 ("disabled index (col)"), new element=w565) -> (w560:string[][])  [unwired: 1 in]
      }
      n142 = Build Array("Instrument Name " ("string"), "Channel Name" ("element"), "Instrument Channel Number" ("element"), "Vertical Range (V)" ("element"), "Vertical Coupling" ("element"), "Min Record Length" ("element"), "Actual Sample Rate" ("element")) -> (w479:string[])
      n143 = Insert Into Array(array=w452, index (col)=0 ("disabled index (col)"), new element=w479) -> (w472:string[][])  [unwired: 1 in]
      n144 = Build Path(base path=w421, name or relative path="Oscilloscope_Params.csv") -> (appended path=w477:path)
      n145 = call-poly <vilib>:"Write Delimited Spreadsheet.vi"("file path (dialog if empty)"=w477, "format (%s)"="%s" ("format (%.3f)"), "2D data"=w472, "error in (no error)"=w475, "transpose? (no:F)"=TRUE, "delimiter (\\t)"="," ("delimiter (\\t)")) -> ("error out"=w470:errorcluster)  [unwired: 8 in, 1 out]
      n146 = for {
        shift-right: [w542] -> w468
        shift-left: string[][] [] ("DCPowerInfoArray") -> [w543]
        tunnel: w458 -> [w558] mode=indexing
        shift-right: [w527] -> w444
        shift-left: w470 -> [w534]
        shift-right: [w535] -> w451
        shift-left: w452 -> [w535]
        shift-right: [w536] -> w453
        shift-left: w454 -> [w536]
        shift-right: [w537] -> w455
        shift-left: w456 -> [w537]
        shift-right: [w538] -> w457
        shift-left: w458 -> [w538]
        shift-right: [w539] -> w443
        shift-left: w459 -> [w539]
        shift-right: [w540] -> w460
        shift-left: w461 -> [w540]
        shift-right: [w541] -> w462
        shift-left: w463 -> [w541]
        n147 = Unbundle(w558) -> ("VISA resource name"=w557:refnum<visa-resource-name>, "Frequency (GHz) Output"=w551:dbl, "Power (dBm) Output"=w548:dbl)  [unwired: 2 out]
        n148 = Decimal String To Number(string="8") -> (number=w546:i32)  [unwired: 2 in, 1 out]
        n149 = VISA Write(VISA resource name=w557, write buffer="*IDN?", error in (no error)=w534) -> (VISA resource name out=w553:refnum<visa-resource-name>, return count=w555:u32, error out=w559:errorcluster)
        n150 = Number To Fractional String(number=w548, precision (6)=w546) -> (F-format string=w549:string)  [unwired: 2 in]
        n151 = Add(x=w555, y=u32 10) -> (x+y=w552:u32)
        n152 = Number To Fractional String(number=w551, precision (6)=w546) -> (F-format string=w550:string)  [unwired: 2 in]
        n153 = VISA Read(VISA resource name=w553, byte count=w552, error in (no error)=w559) -> (read buffer=w533:string, error out=w528:errorcluster)  [unwired: 2 out]
        n154 = Search and Replace String(replace all?=TRUE ("replace all? (F)"), input string=w533, search string=",", replace string="_" ("replace string (\"\")"), error in=w528) -> (result string=w530:string, error out=w527:errorcluster)  [unwired: 3 in, 2 out]
        n155 = Build Array(w530, w550, w549) -> (w545:string[])
        n156 = Insert Into Array(array=w543, index (col)=0 ("index (row)"), new element=w545) -> (w542:string[][])  [unwired: 1 in]
      }
      n157 = Build Array("Instrument Name", "Frequency (GHz)" ("element"), "Power (dBm)" ("element")) -> (w464:string[])
      n158 = Insert Into Array(array=w468, index (col)=0 ("disabled index (col)"), new element=w464) -> (w445:string[][])  [unwired: 1 in]
      n159 = Build Path(base path=w421, name or relative path="RFSource_Params.csv") -> (appended path=w449:path)
      n160 = call-poly <vilib>:"Write Delimited Spreadsheet.vi"("file path (dialog if empty)"=w449, "format (%s)"="%s" ("format (%.3f)"), "2D data"=w445, "error in (no error)"=w444, "transpose? (no:F)"=TRUE, "delimiter (\\t)"="," ("delimiter (\\t)")) -> ("error out"=w424:errorcluster)  [unwired: 8 in, 1 out]
      n161 = Strip Path(path=w421) -> (name=w442:string)  [unwired: 1 out]
      n162 = Unbundle(w443) -> ("DUT"=w441:string, "Ion (ex Kr)"=w440:string, "Board Number"=w439:string, "Effective LET"=w438:string, "Test Type"=w437:T13)  [unwired: 1 out]
      n163 = case shown="\"Single Event Latchup\", Default" w437 {
        tunnel: ["Single Event Latchup (SEL)" "Single Event Transient (SET)"] -> w436
        frame "Single Event Latchup", Default {
        }
        frame "Single Event Transient" {
        }
      }
      n164 = Build Array("Run Number" ("name"), "DUT" ("element"), "Ion" ("element"), "Board Number" ("element"), "Effective LET" ("element"), "Test Type" ("element")) -> (w435:string[])
      n165 = Build Array(w442, w441, w440, w439, w438, w436) -> (w434:string[])
      n166 = Build Array(w435, w434) -> (w422:string[][])
      n167 = Build Path(base path=w421, name or relative path="RunData_Params.csv") -> (appended path=w429:path)
      n168 = call-poly <vilib>:"Write Delimited Spreadsheet.vi"("file path (dialog if empty)"=w429, "format (%s)"="%s" ("format (%.3f)"), "2D data"=w422, "error in (no error)"=w424, "transpose? (no:F)"=TRUE, "delimiter (\\t)"="," ("delimiter (\\t)")) -> ("error out"=w423:errorcluster)  [unwired: 8 in, 1 out]
    }
  }
  "DCPowerInformationClusterArray_Output" <- w41
  "VISAPowerInfoInputOutput" <- w43
  "Run Data SubPanel Output" <- w45
  "RF Block Parameters Output" <- w47
  "Oscilloscope Info Array Output" <- w49
  "Data Was Collected?" <- w38
  "DCPowerInfoArray" <- w37
  "OscilloscopeInfoArray" <- w3
  "RFSourceInfoArray" <- w2
  n169 = List Folder(path=w35, pattern="*.txt", error in=w53) -> (path out=w58:path, filenames=w57:string[], error out=w56:errorcluster)  [unwired: 1 in, 1 out]
  n170 = for {
    tunnel: [w619] -> w6
    tunnel: w58 -> [w619]
    tunnel: w57 -> [w621] mode=indexing
    shift-right: [w622] -> w21
    shift-left: w56 -> [w623]
    n171 = Build Path(base path=w619, name or relative path=w621) -> (appended path=w620:path)
    n172 = Delete(path (use dialog)=w620, error in=w623) -> (error out=w622:errorcluster)  [unwired: 3 in, 2 out]
  }
  n173 = Get Date/Time String(date format (0)=enum16{"short", "long", "abbreviated"}."short", seconds (now)=w19, want seconds? (F)=TRUE) -> (date string=w14:string, time string=w15:string)
  n174 = Concatenate Strings(w14, "," ("string"), w15) -> (w13:string)
  n175 = Strip Path(path=w6) -> (name=w62:string)  [unwired: 1 out]
  n176 = Build Path(base path=w6, name or relative path="BeginRecordTimeStamp.txt") -> (appended path=w5:path)
  n177 = Concatenate Strings(w62, "_DCPOWER_COPYFOLDER" ("name or relative path")) -> (w60:string)
  n178 = Open/Create/Replace File(file path (use dialog)=w5, error in=w21, operation (0:open)=T8."open or create", access (0:read/write)=enum16{"read/write", "read-only", "write-only"}."read/write") -> (refnum out=w12:refnum<file>, error out=w20:errorcluster)  [unwired: 2 in, 1 out]
  n179 = Build Path(base path=w6, name or relative path=w60) -> (appended path=w69:path)
  n180 = Write to Text File(file (use dialog)=w12, text=w13, error in=w20) -> (refnum out=w8:refnum<file>, error out=w9:errorcluster)  [unwired: 1 in, 1 out]
  n181 = Close File(refnum=w8, error in=w9) -> (error out=w7:errorcluster)  [unwired: 1 out]
  n182 = Create Folder(path (use dialog)=w69, error in=w7) -> (created path=w64:path, error out=w67:errorcluster)  [unwired: 1 in, 1 out]
  n183 = List Folder(path=w6, error in=w67) -> (path out=w66:path, filenames=w65:string[], error out=w63:errorcluster)  [unwired: 2 in, 1 out]
  n184 = for {
    tunnel: w66 -> [w629]
    tunnel: w65 -> [w628] mode=indexing
    tunnel: w64 -> [w624]
    shift-right: [w631] -> w68
    shift-left: w63 -> [w625]
    tunnel: [w624] -> _
    n185 = Build Path(base path=w629, name or relative path=w628) -> (appended path=w626:path)
    n186 = Build Path(base path=w624, name or relative path=w628) -> (appended path=w627:path)
    n187 = Copy(8:w625, 9:TRUE ("overwrite (F)"), 10:w627, 11:w626) -> (0:w631:errorcluster)  [unwired: 1 in, 2 out]
  }
  "error out" <- w68
